vi "GPIB Address Check.vi"(0 "Instrument Address":refnum<visa-resource-name>, 1 "Term Char":string) -> (2 "dup VISA session":refnum<visa-resource-name>, 3 "status":u16, 4 "error out":errorcluster)   [LabVIEW 2020]
doc: "Checks the status of a device on the GPIB bus. If it is a listener then it is requested to return a status byte. Both checks are done since a GPIB isolator can fool this because it is a listener at all addresses but will not return a status byte.\nScott Hannahs, <sth@magnet.fsu.edu> NHMFL-FSU, May 2003"
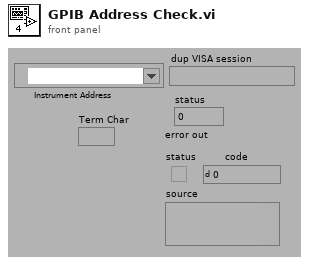
[diagram p1: front panel]
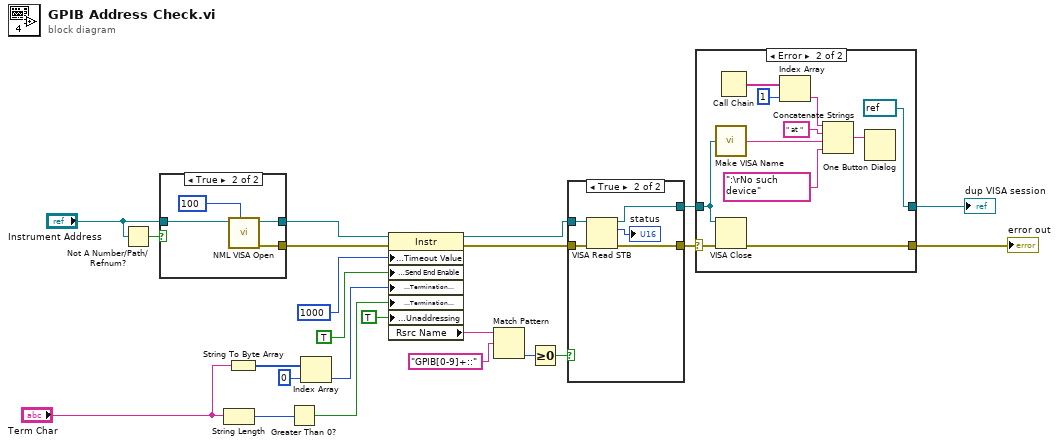
[diagram p0: block diagram]
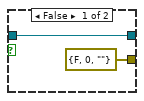
[diagram p2: hidden frame]
diagram:
  n1 = Not A Number/Path/Refnum?(number/path/refnum="Instrument Address") -> (NaN/Path/Refnum?=w6:bool)
  n2 = case shown="True" w6 {
    tunnel: "Instrument Address" -> [w25 w28]
    tunnel: [w25 w27] -> w3
    tunnel: [errorcluster {"status"=FALSE, "code"=0, "source"=""} ("error out") w26] -> w2
    frame False {
    }
    frame True {
      n3 = call "NML VISA Open.vi"("VISA Open timeout (0)"=u32 100, "VISA resource name"=w28) -> ("error out"=w26:errorcluster, "VISA resource name out"=w27:refnum<visa-resource-name>)  [unwired: 8 in]
    }
  }
  n4 = String Length(string="Term Char") -> (length=w17:i32)
  n5 = String To Byte Array(string="Term Char") -> (unsigned byte array=w23:u8[])
  n6 = Greater Than 0?(x=w17) -> (x > 0?=w16:bool)
  n7 = Index Array(array=w23, index=0 ("Index")) -> (element=w21:u8)
  n8 = property class="Instr"(reference=w3, error in=w2, "General Settings:Timeout Value"=u32 1000, "Message Based Settings:Send End Enable"=TRUE, "Message Based Settings:Termination Character"=w21, "Message Based Settings:Termination Character Enable"=w16, "GPIB Settings:Unaddressing"=TRUE ("GPIB Settings:GPIB Unaddressing")) -> (reference out=w15:refnum<visa-resource-name>, error out=w14:errorcluster, "Rsrc Name"=w5:string)
  n9 = Match Pattern(string=w5, regular expression="GPIB[0-9]+::") -> (offset past match=w9:i32)  [unwired: 1 in, 3 out]
  n10 = Greater Or Equal To 0?(x=w9) -> (x >= 0?=w8:bool)
  n11 = case shown="True" w8 {
    tunnel: w15 -> [w31 w36]
    tunnel: w14 -> [w30 w35]
    tunnel: [w31 w33] -> w13
    tunnel: [w30 w32] -> w1
    frame False {
    }
    frame True {
      n12 = VISA Read STB(8:w35, 11:w36) -> (0:w32:errorcluster, 2:→"status":u16, 3:w33:refnum<visa-resource-name>)
    }
  }
  n13 = case shown="Error" w1 {
    selector: w1 -> [w37 w39]
    tunnel: w13 -> [w38 w40]
    tunnel: [w37 w47] -> w12
    tunnel: [w38 refnum<visa-resource-name> refnum ("dup VISA session")] -> w11
    frame No Error {
    }
    frame Error {
      n14 = call "Make VISA Name.vi"("Instrument Address"=w40) -> ("Name"=w41:string)
      n15 = VISA Close(VISA resource name=w40, error in (no error)=w39) -> (error out=w47:errorcluster)
      n16 = Call Chain() -> (call chain=w48:string[])
      n17 = Index Array(array=w48, index=1) -> (element=w43:string)
      n18 = Concatenate Strings(w43, " at ", w41, ":\rNo such device") -> (w45:string)
      n19 = One Button Dialog(message=w45) -> ()  [unwired: 1 in, 1 out]
    }
  }
  "error out" <- w12
  "dup VISA session" <- w11
